vi "Clear Timing Override.vi"(8 "error in (no error)":errorcluster, 10 "Clear Timing Override":bool, 11 "CIFTemplateNode in":refnum<class "CIFCorePlugin.lvclass">) -> (0 "error out":errorcluster, 3 "CIFTemplateNode out":refnum<class "CIFCorePlugin.lvclass">)   [LabVIEW 2021, in "CIFCorePlugin.lvclass"]
uses:
  CIFCorePlugin.lvclass
  CIFCorePlugin.lvclass/CIFCorePlugin.ctl
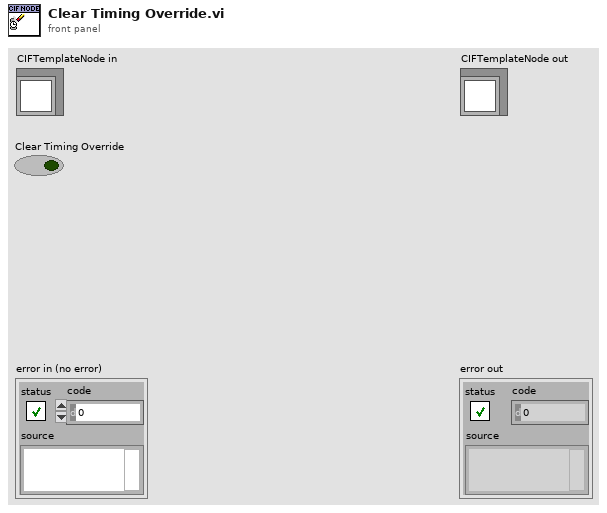
[diagram p1: front panel]
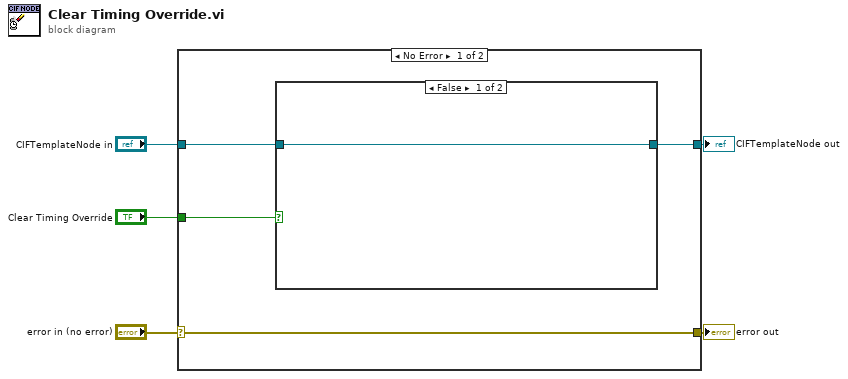
[diagram p0: block diagram]
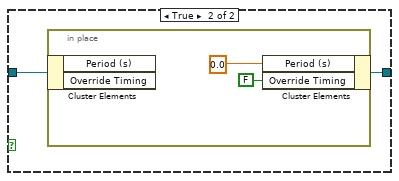
[diagram p2: hidden frame]
diagram:
  n1 = case shown="No Error" "error in (no error)" {
    selector: "error in (no error)" -> [w9 w15]
    tunnel: [w9 w15] -> w4
    tunnel: [w7 w16] -> w2
    tunnel: "CIFTemplateNode in" -> [w8 w16]
    tunnel: "Clear Timing Override" -> [w6 _]
    frame No Error {
      n2 = case shown="False" w6 {
        tunnel: w8 -> [w10 w12]
        tunnel: [w10 w11] -> w7
        frame False {
        }
        frame True {
          n3 = in-place {
            n4 = in-place-cluster #1(w12) -> ()  [unwired: 2 out]
            n5 = in-place-cluster #1("Period (s)"=0.0, "Override Timing"=FALSE ("Plugin Overrides.Timing Overrides.Override Timing")) -> (w11:refnum<class "CIFCorePlugin.lvclass">)
          }
        }
      }
    }
    frame Error {
    }
  }
  "error out" <- w4
  "CIFTemplateNode out" <- w2
